vi "AssertDisabledItems.vi"(0 "VI Reference In":refnum<vi>, 1 "Test Label":string, 2 "delimiter (>>)":string=">>", 3 "Assert Only? (F)":bool, 5 "Control Path":string, 7 "Disabled Items":i32[](array[numeric]), 11 "Error In":errorcluster, 12 "Assert Interval(10 ms)":u32=10, 13 "Timeout(5 sec)":dbl=5.0) -> (4 "VI Reference Out":refnum<vi>, 6 "Asserted Value":i32[](array[numeric]), 15 "Error Out":errorcluster)   [LabVIEW 2016, in "Drona.lvlib" / "AssertControlValue.lvlib" / "AssertListbox.lvlib"]
doc: "Asserts if the disabled items on the listbox control are equal.\n\nThe input control name is given as a string , incase of path, use delimiters inbetween the path.\nThis VI gets the value of the control, untill the value is equal to the input value."
uses:
  AssertListbox.lvlib
  Get/GetControlRef/GetControlRefByPath.vi
  <vilib>/addons/_JKI Toolkits/Caraya/classes/Assert/Assert Equal Value_Variant.vi
  <vilib>/Utility/error.llb/Error Cluster From Error Code.vi
  <vilib>/ErrorRing/Error Ring.xnode
  <vilib>/addons/_JKI Toolkits/Caraya/classes/Assert/Assert.lvclass
  Get/GetControlRef/GetControlRef.lvlib
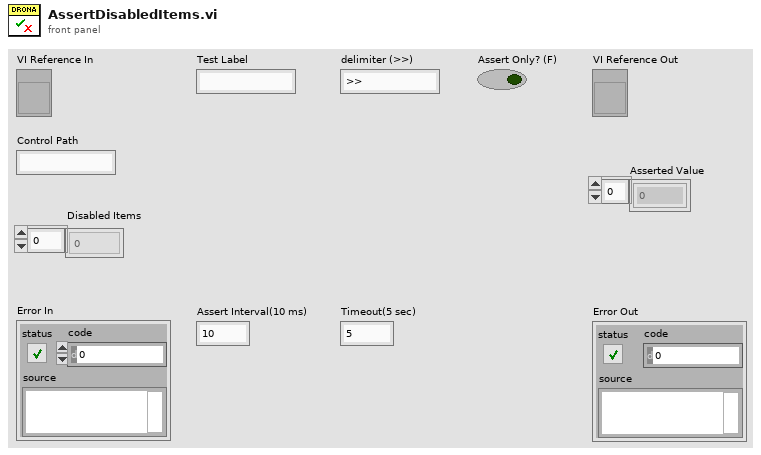
[diagram p1: front panel]
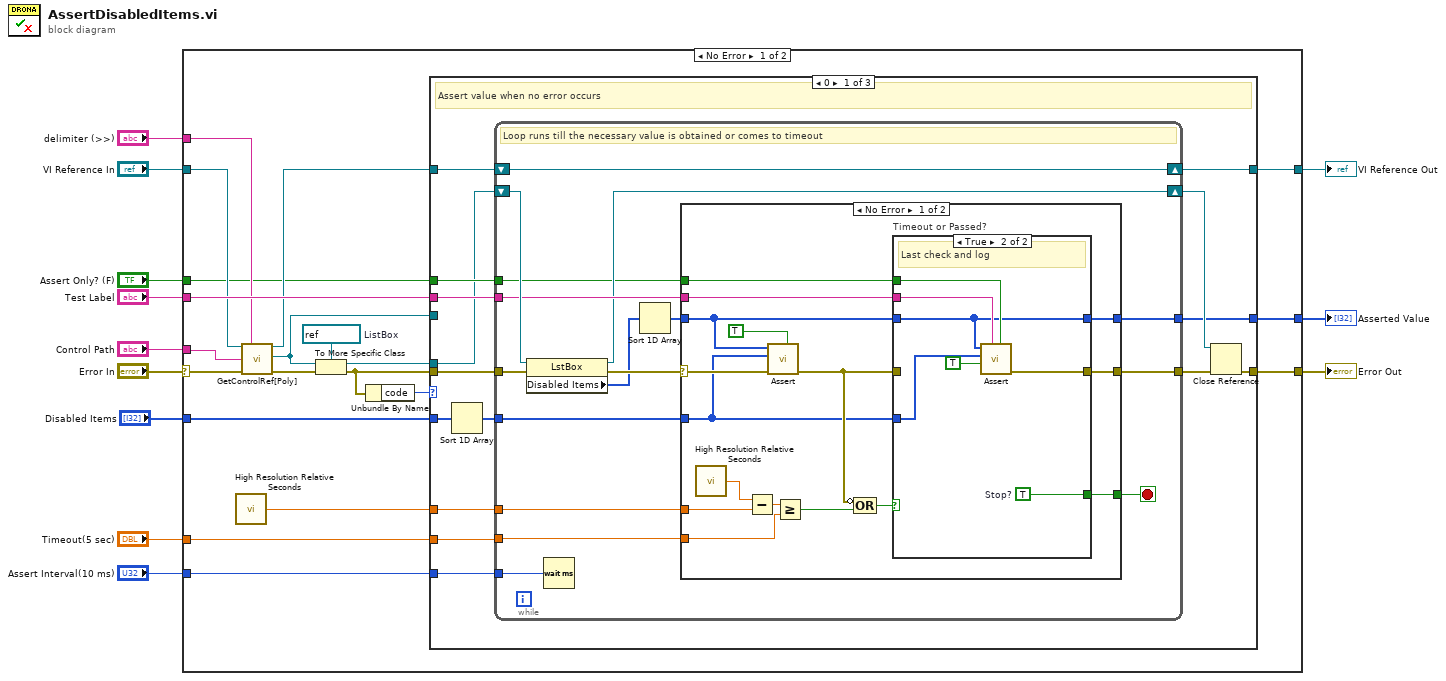
[diagram p0: block diagram]
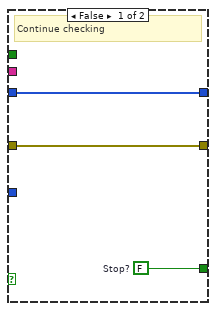
[diagram p2: hidden frame]
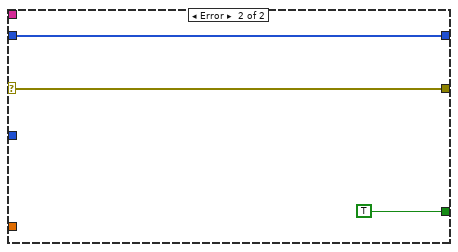
[diagram p3: hidden frame]
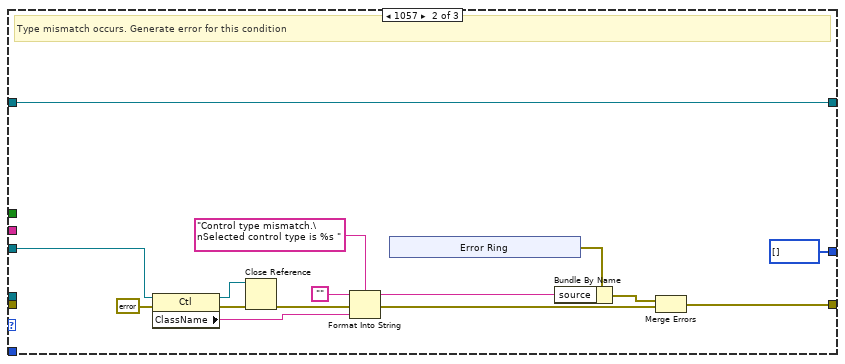
[diagram p4: hidden frame]
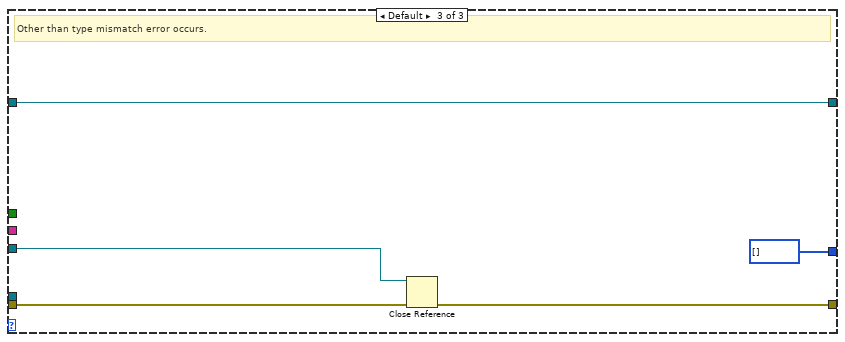
[diagram p5: hidden frame]
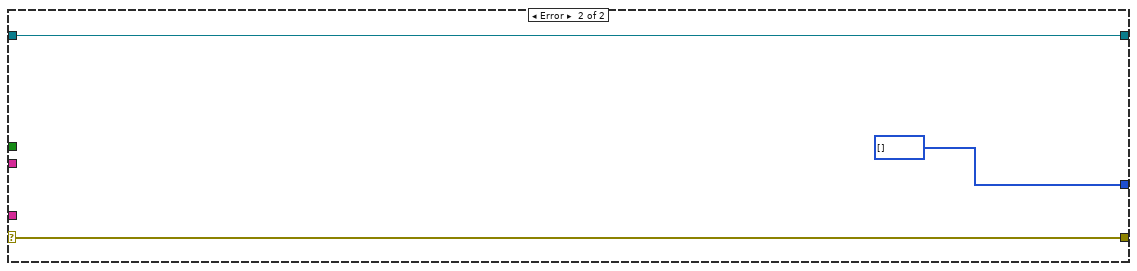
[diagram p6: hidden frame]
diagram:
  n1 = case shown="No Error" "Error In" {
    selector: "Error In" -> [w28 w120]
    tunnel: "Timeout(5 sec)" -> [w32 _]
    tunnel: [w31 w119] -> w11
    tunnel: [w22 w120] -> w10
    tunnel: "Assert Interval(10 ms)" -> [w30 _]
    tunnel: "Test Label" -> [w29 _]
    tunnel: "VI Reference In" -> [w27 w119]
    tunnel: "Control Path" -> [w26 _]
    tunnel: "delimiter (>>)" -> [w21 _]
    tunnel: "Assert Only? (F)" -> [w20 _]
    tunnel: [w19 i32[] []] -> w1
    tunnel: "Disabled Items" -> [w16 _]
    frame No Error {
      w18 = refnum<vi> refnum  # ListBox
      n2 = call <vilib>:"High Resolution Relative Seconds.vi"() -> ("relative seconds"=w25:dbl)
      n3 = call-poly "GetControlRef[Poly].vi"("VI Reference In"=w27, "delimiter (>>)"=w21, "Control Path"=w26, "error In"=w28) -> ("VI Reference Out"=w23:refnum<vi>, "Ctl Refnum"=w13:refnum<vi>, "error out"=w24:errorcluster)  [unwired: 9 in]
      n4 = To More Specific Class(target class=w18, reference=w13, error in=w24) -> (specific class reference=w17:refnum<vi>, error out=w15:errorcluster)
      n5 = Unbundle By Name(w15) -> ("code"=w14:i32)
      n6 = case shown="0" w14 {
        tunnel: w32 -> [w47 _ _]
        tunnel: [w46 w93 w117] -> w31
        tunnel: w30 -> [w44 _ _]
        tunnel: w29 -> [w43 _ _]
        tunnel: w25 -> [w42 _ _]
        tunnel: w23 -> [w41 w93 w117]
        tunnel: [w40 w96 w114] -> w22
        tunnel: w20 -> [w38 _ _]
        tunnel: [w37 i32[] [] i32[] []] -> w19
        tunnel: w15 -> [w36 _ w115]
        tunnel: w17 -> [w35 _ _]
        tunnel: w16 -> [w34 _ _]
        tunnel: w13 -> [_ w95 w113]
        frame 0 {
          # "Assert value when no error occurs"
          n7 = Sort 1D Array(array=w34) -> (sorted array=w33:i32[])
          n8 = while {
            tunnel: w47 -> [w62]
            tunnel: w42 -> [w63]
            tunnel: w36 -> [w57]
            tunnel: [w60] -> w45
            tunnel: w44 -> [w58]
            tunnel: w43 -> [w54]
            shift-right: [w55] -> w46
            shift-left: w41 -> [w55]
            shift-right: [w53] -> w39
            shift-left: w35 -> [w56]
            tunnel: w38 -> [w52]
            tunnel: [w51] -> w37
            tunnel: w33 -> [w50]
            stop <- w61 stop-if-true
            # "Loop runs till the necessary value is obtained or comes to timeout"
            n9 = property on="Property Node" class="LstBox"(reference=w56, error in=w57) -> (reference out=w53:refnum<vi>, error out=w59:errorcluster, "Disabled Items"=w49:i32[])
            n10 = Wait (ms)(milliseconds to wait=w58) -> ()  [unwired: 1 out]
            n11 = Sort 1D Array(array=w49) -> (sorted array=w48:i32[])
            n12 = case shown="No Error" w59 {
              selector: w59 -> [w75 w92]
              tunnel: w63 -> [w79 _]
              tunnel: w62 -> [w76 _]
              tunnel: [w67 TRUE] -> w61
              tunnel: [w68 w92] -> w60
              tunnel: w48 -> [w69 w90]
              tunnel: w54 -> [w74 _]
              tunnel: w52 -> [w66 _]
              tunnel: [w65 w90] -> w51
              tunnel: w50 -> [w64 _]
              frame No Error {
                n13 = call <vilib>:"High Resolution Relative Seconds.vi"() -> ("relative seconds"=w78:dbl)
                n14 = Subtract(x=w78, y=w79) -> (x-y=w77:dbl)
                n15 = call-poly <vilib>:"Assert.vi"("Assert Only? (F)"=TRUE, "error in (no error)"=w75, "Y"=w64, "X"=w69) -> ("error out"=w72:errorcluster)  [unwired: 7 in]
                n16 = Greater Or Equal?(x=w77, y=w76) -> (x >= y?=w73:bool)
                n17 = Compound Arithmetic op=OR(invert w72, w73) -> (w71:bool)
                n18 = case "Timeout or Passed?" shown="True" w71 {
                  tunnel: w72 -> [w82 _]
                  tunnel: w69 -> [w80 w84]
                  tunnel: w74 -> [_ w89]
                  tunnel: [w82 w88] -> w68
                  tunnel: [w81 w87] -> w67
                  tunnel: w66 -> [_ w85]
                  tunnel: [w80 w84] -> w65
                  tunnel: w64 -> [_ w83]
                  frame False {
                    w81 = FALSE  # Stop?
                    # "Continue checking"
                  }
                  frame True {
                    w87 = TRUE  # Stop?
                    # "Last check and log"
                    n19 = call-poly <vilib>:"Assert.vi"("Assert Only? (F)"=w85, "Label"=w89, "Register with caller test (F)"=TRUE, "Y"=w83, "X"=w84) -> ("error out"=w88:errorcluster)  [unwired: 6 in]
                  }
                }
              }
              frame Error {
              }
            }
          }
          n20 = Close Reference(reference=w39, error in (no error)=w45) -> (error out=w40:errorcluster)
        }
        frame 1057 {
          # "Type mismatch occurs. Generate error for this condition"
          n21 = property class="Ctl"(reference=w95, error in=errorcluster {"status"=FALSE, "code"=0, "source"=""} ("error out")) -> (reference out=w97:refnum<vi>, error out=w107:errorcluster, "ClassName"=w104:string)
          n22 = Close Reference(reference=w97, error in (no error)=w107) -> (error out=w98:errorcluster)
          n23 = Format Into String(format string="Control type mismatch.\nSelected control type is %s ", initial string="", error in=w98, w104) -> (resulting string=w101:string, error out=w99:errorcluster)
          n24 = xnode "Error Ring"() -> ("error out"=w102:errorcluster)
          n25 = Bundle By Name(cluster=w102, "source"=w101) -> (w100:errorcluster)
          n26 = Merge Errors(w100, w99) -> (w96:errorcluster)
        }
        frame Default {
          # "Other than type mismatch error occurs."
          n27 = Close Reference(reference=w113, error in (no error)=w115) -> (error out=w114:errorcluster)
        }
      }
    }
    frame Error {
    }
  }
  "Error Out" <- w10
  "VI Reference Out" <- w11
  "Asserted Value" <- w1
